vi "Write LUT.vi"(8 "error in (no error)":errorcluster, 10 "LUT":variant, 11 "ObjectLUT in":refnum<class "ObjectLUT.lvclass">) -> (0 "error out":errorcluster, 3 "ObjectLUT out":refnum<class "ObjectLUT.lvclass">)   [LabVIEW 2020, in "ORM_lib.lvlib" / "ObjectLUT.lvclass"]
uses:
  ObjectLUT.lvclass
  ObjectLUT.lvclass/ObjectLUT.ctl
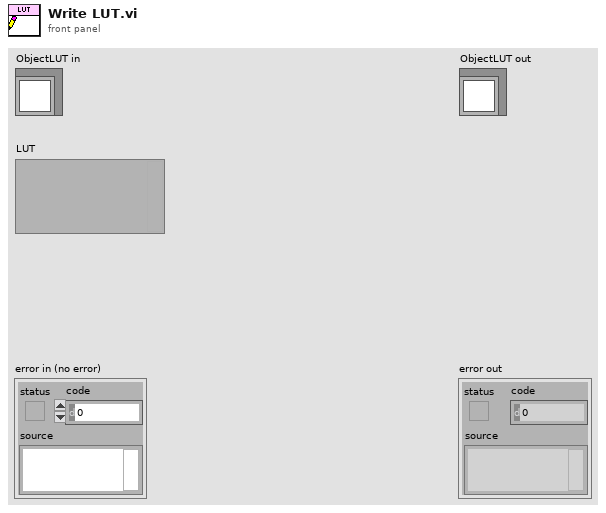
[diagram p1: front panel]
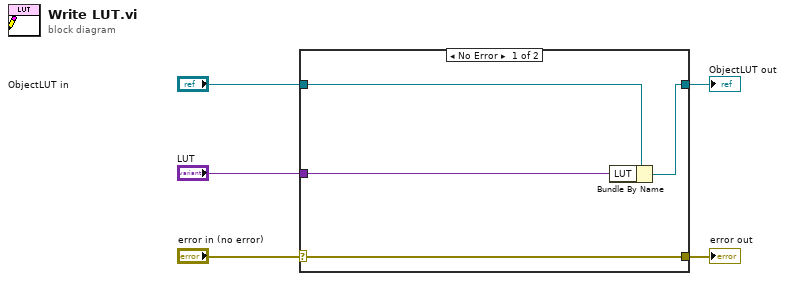
[diagram p0: block diagram]
diagram:
  n1 = case shown="No Error" "error in (no error)" {
    selector: "error in (no error)" -> [w9 w10]
    tunnel: [w9 w10] -> w4
    tunnel: [w7 w11] -> w2
    tunnel: "ObjectLUT in" -> [w8 w11]
    tunnel: "LUT" -> [w6 _]
    frame No Error {
      n2 = Bundle By Name(cluster=w8, "LUT"=w6) -> (w7:refnum<class "ObjectLUT.lvclass">)
    }
    frame Error {
    }
  }
  "error out" <- w4
  "ObjectLUT out" <- w2
